vi "Main.vi"() -> ()   [LabVIEW 2020]
panel:
  out "Postać kanoniczna":string
  out "Max":dbl
  out "Min":dbl
  in  "Rząd pochodnej":i32=1 min=1 max=100
  out "string":string
  out "q":dbl
  out "p":dbl
  in  "start":dbl
  in  "end":dbl
  out "x3":string
  out "x2":string
  out "x1":string
  in  "równanie":bool
  in  "pochodna":bool
  in  "Liczby zespolone":bool
  out "Wykres":cluster{"Xaxis":dbl[], "f'(x)":dbl[]}[](graph)
  in  "x":dbl
  in  "f(x)":bool
  out "Wartość f(x)":dbl
  in  "stop":bool
  in  "d":dbl
  in  "c":dbl
  in  "b":dbl
  in  "a":dbl
  # "Podaj współczynniki:"
  # "Postać wzoru do podania: \n\nax^3 + bx^2 +cx +d =0"
  # "Zakres:"
  # "Współrzędne wierzchołka"
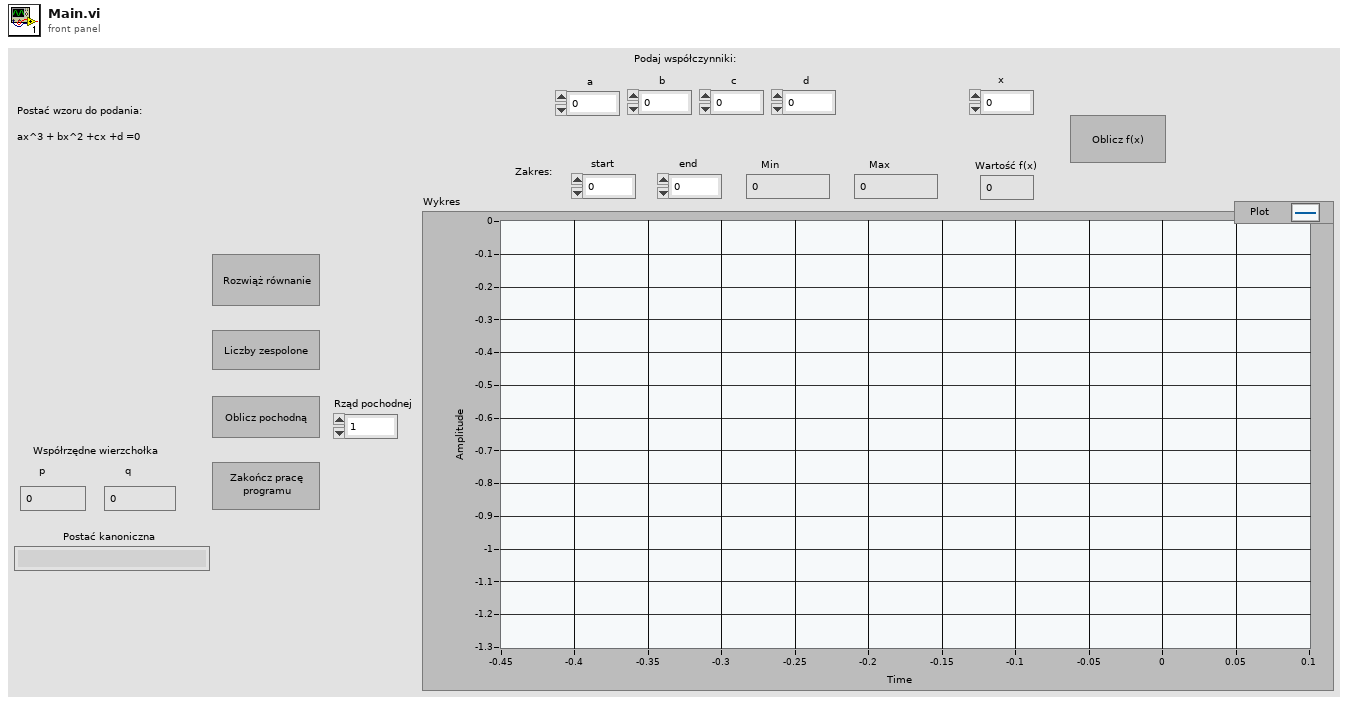
[diagram p1: front panel]
types:
  T1 = cluster{"współczynniki":cluster{"a":dbl, "b":dbl, "c":dbl, "d":dbl}, "x":dbl, "dFx":dbl[], "x2":cdb, "x3":cdb, "wsp. dFx":dbl[], "zespolone?":bool, "p":dbl, "q":dbl, "x[]":dbl[], "zakres":cluster{"od":dbl, "do":dbl}, "x1":cdb, "f(x)":dbl[], "stopień":enum16{"2", "3"}, "delta":i16, "Postać kanoniczna":string}
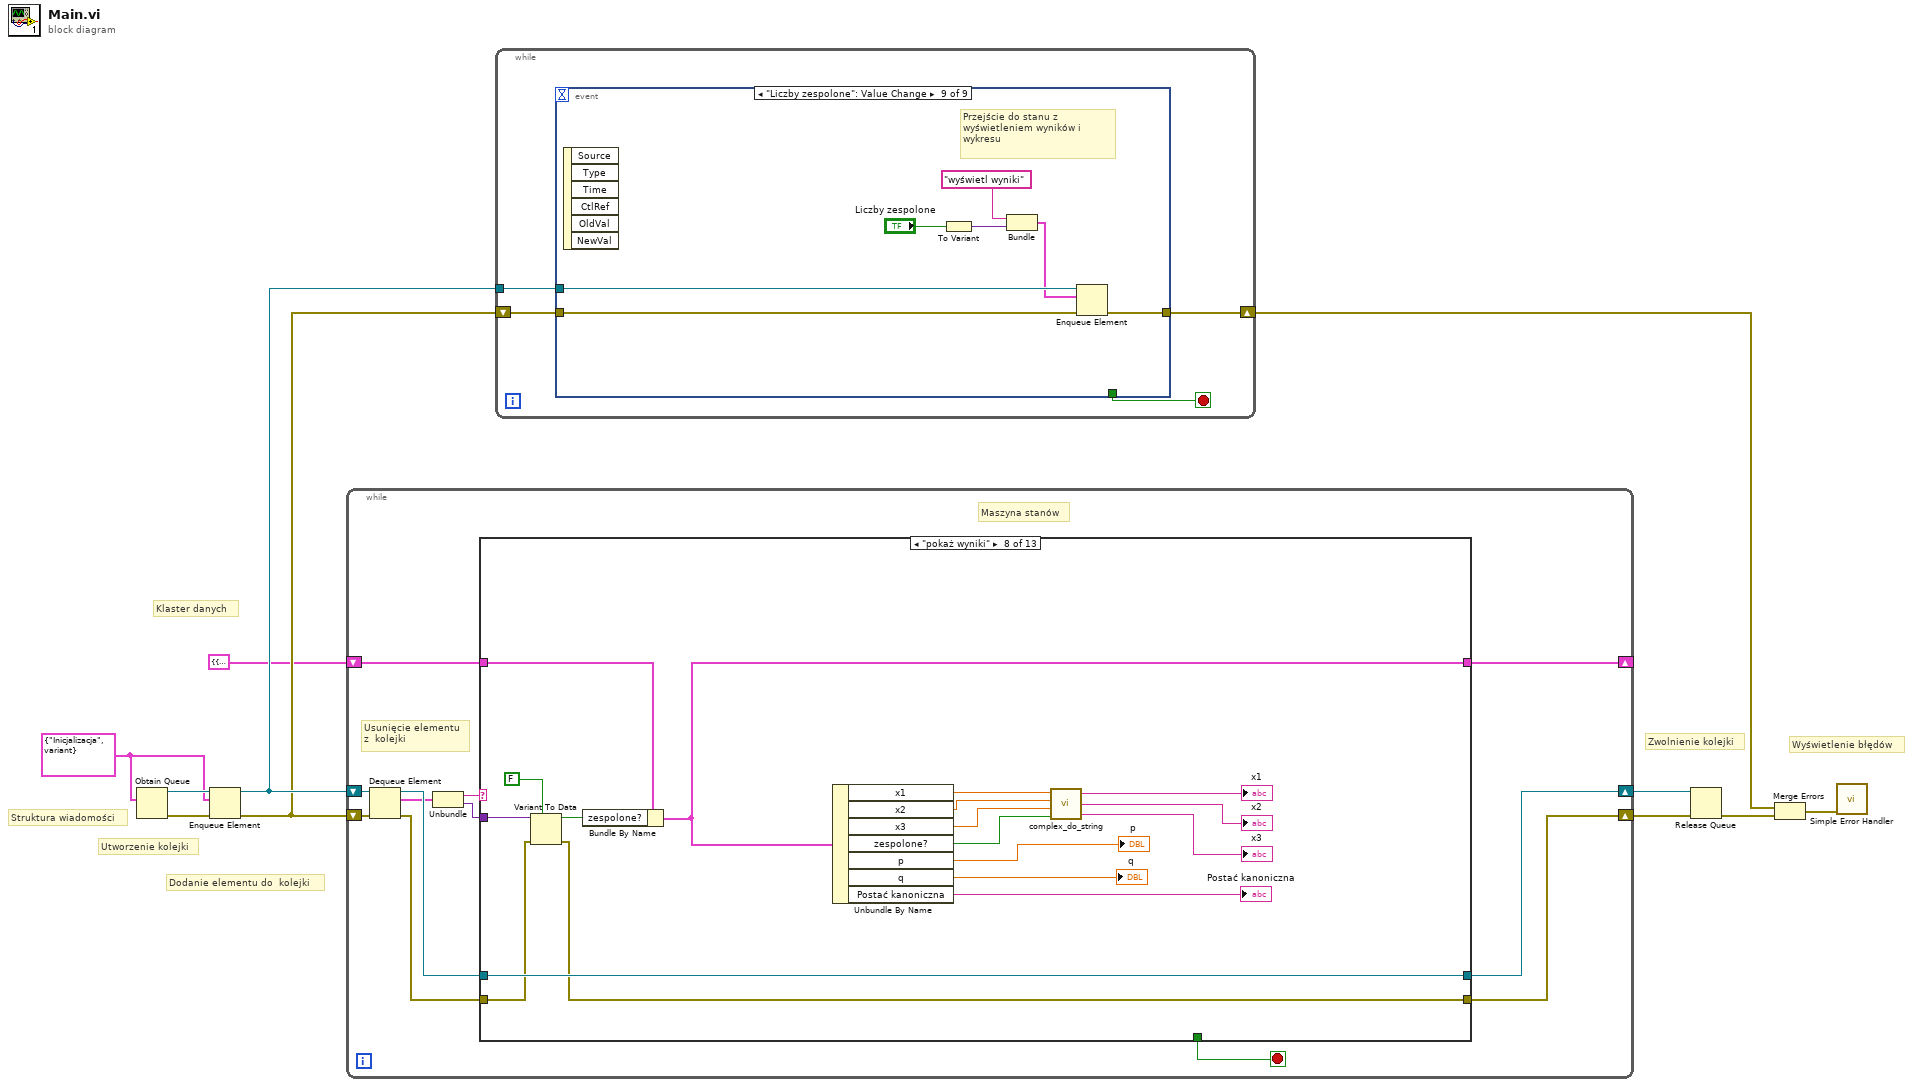
[diagram p0: block diagram]
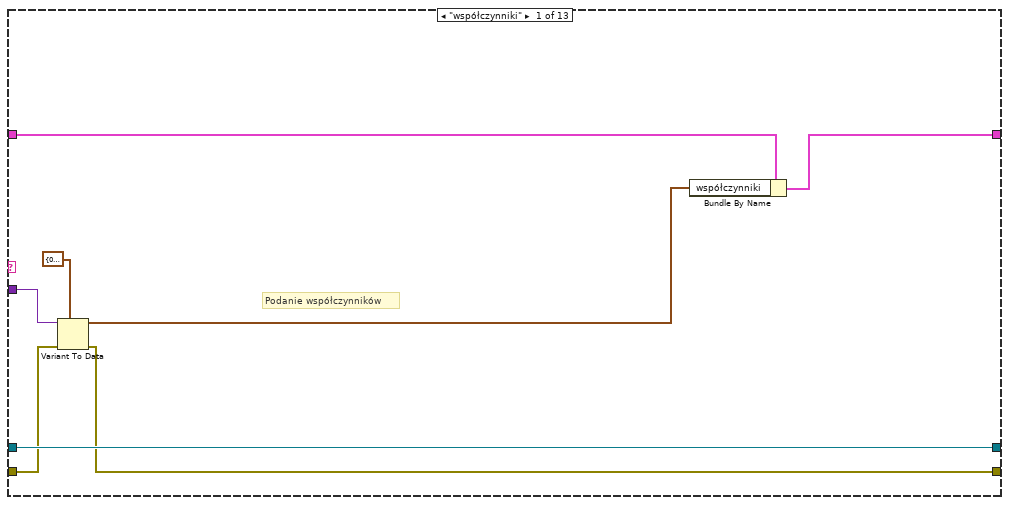
[diagram p2: hidden frame]
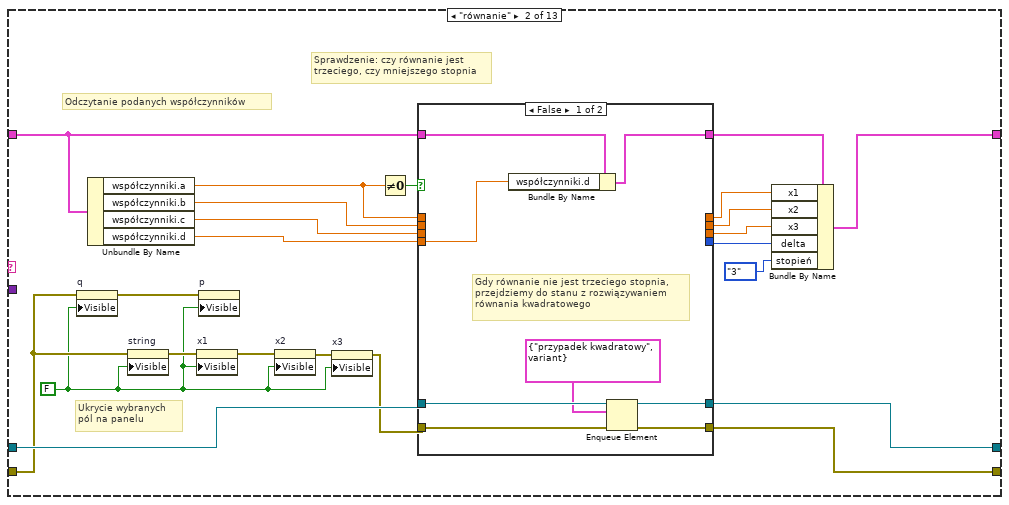
[diagram p3: hidden frame]
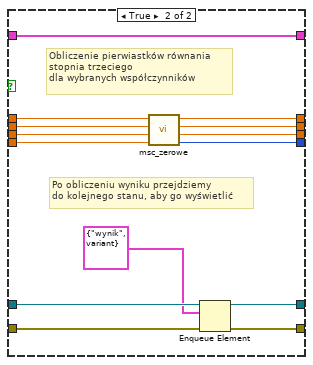
[diagram p4: hidden frame]
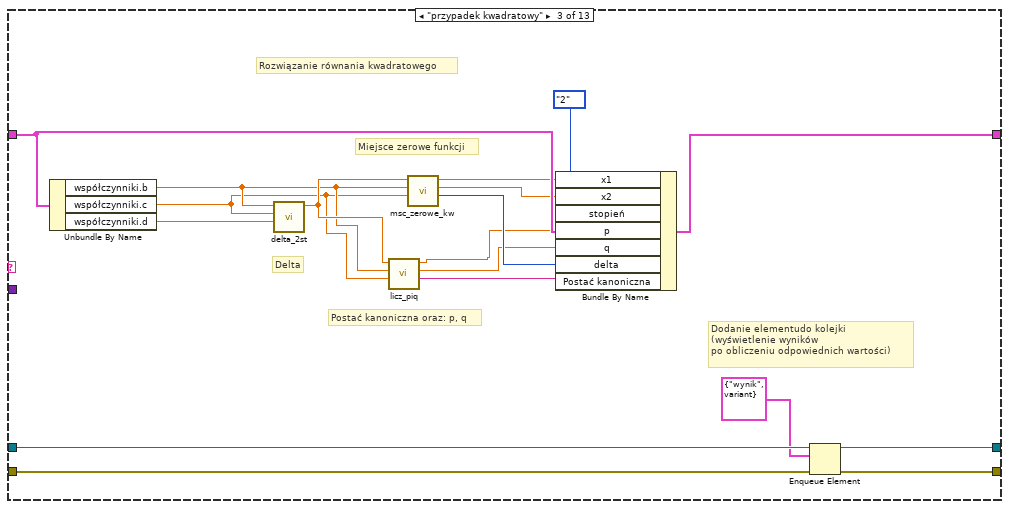
[diagram p5: hidden frame]
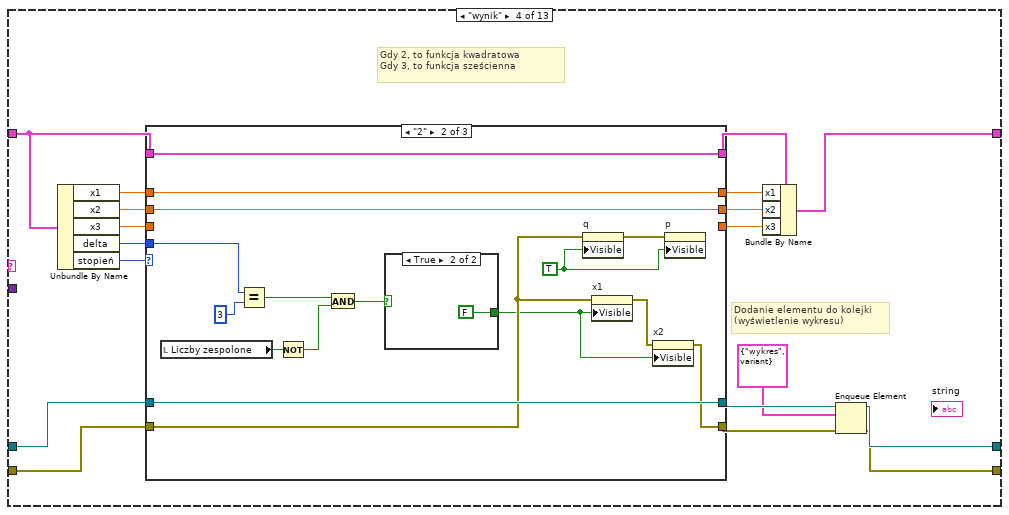
[diagram p6: hidden frame]
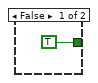
[diagram p8: hidden frame]
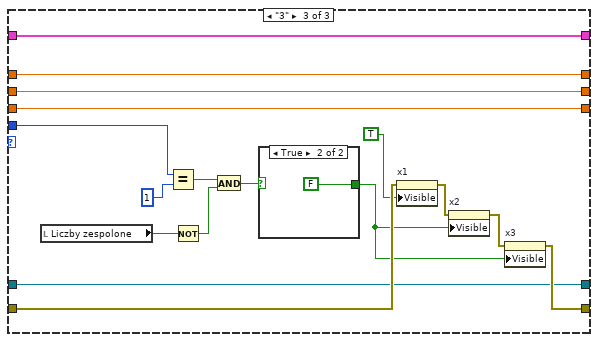
[diagram p9: hidden frame]
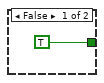
[diagram p10: hidden frame]
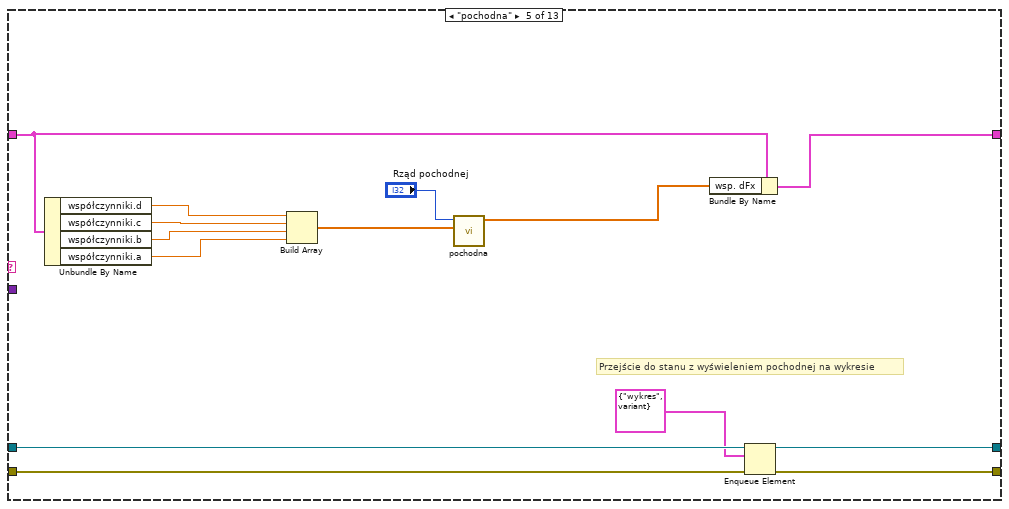
[diagram p11: hidden frame]
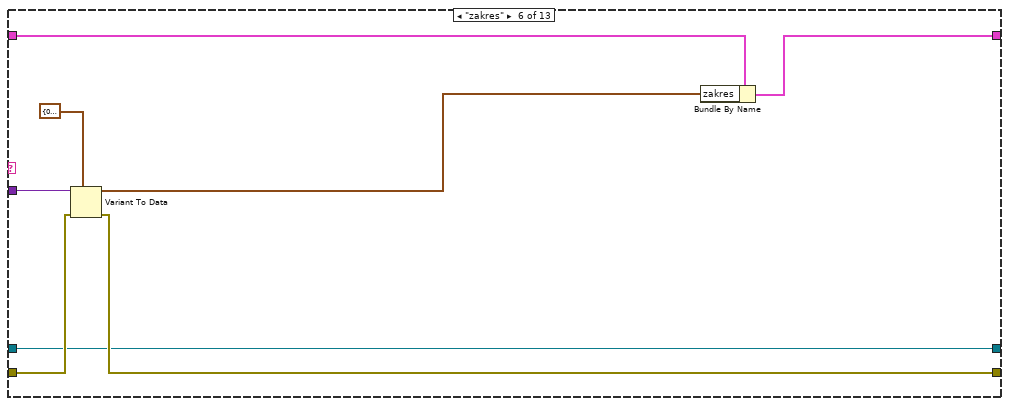
[diagram p12: hidden frame]
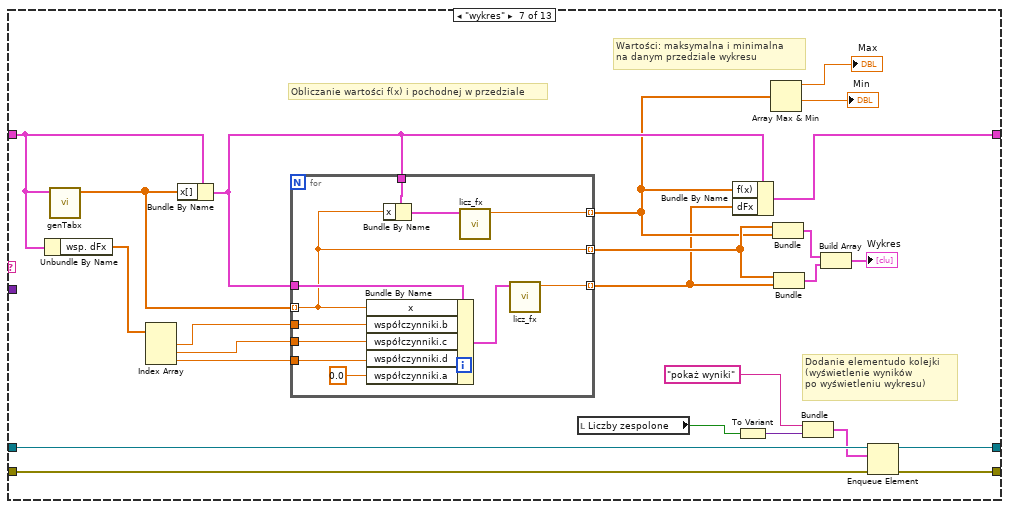
[diagram p13: hidden frame]
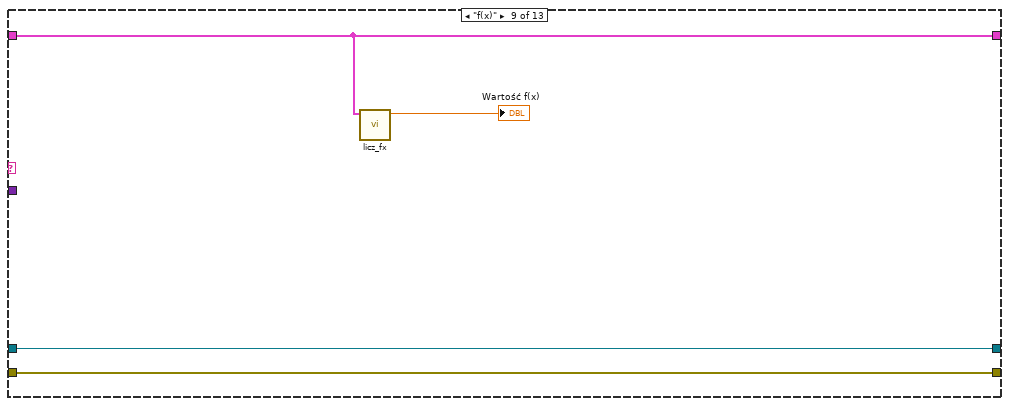
[diagram p14: hidden frame]
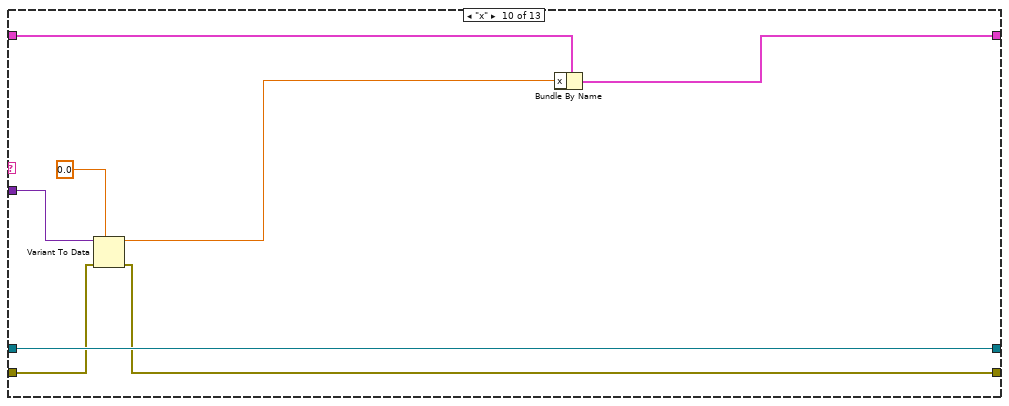
[diagram p15: hidden frame]
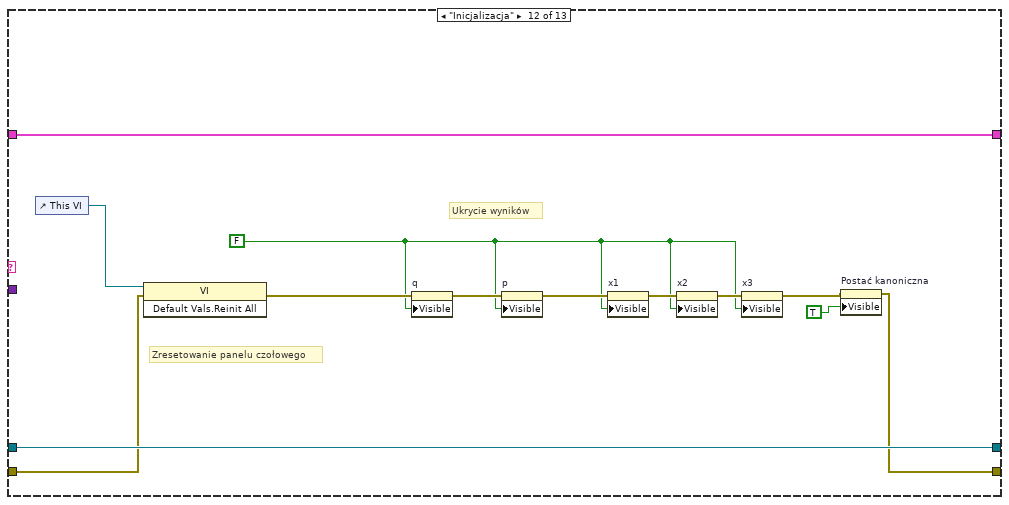
[diagram p17: hidden frame]
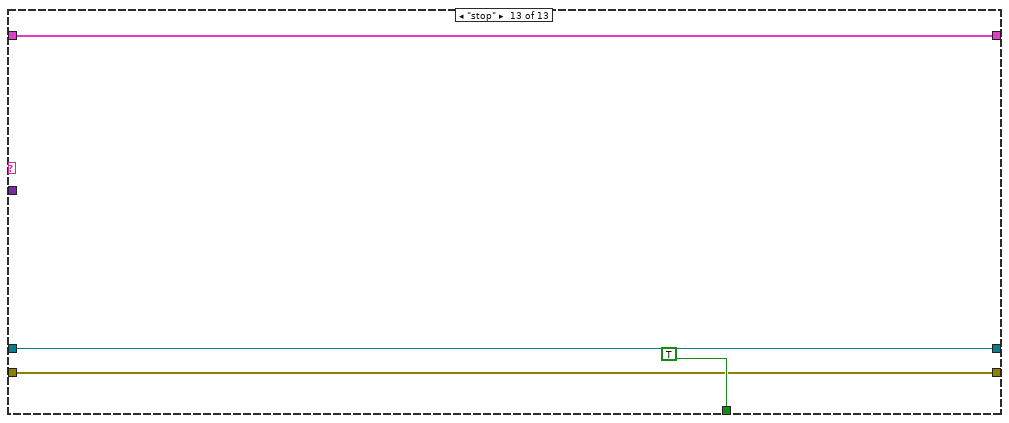
[diagram p18: hidden frame]
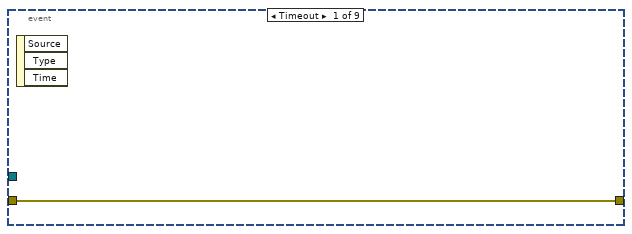
[diagram p19: hidden frame]
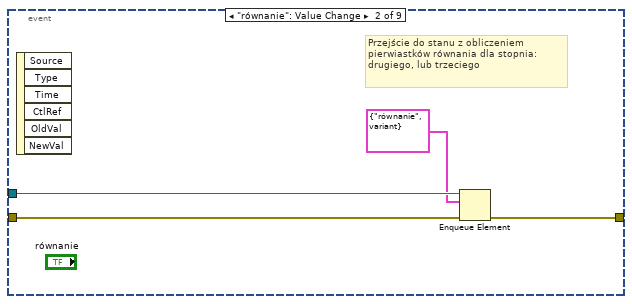
[diagram p20: hidden frame]
diagram:
  w9 = cluster{string, variant} {"Inicjalizacja", variant}
  # "Dodanie elementu do  kolejki"
  # "Struktura wiadomości"
  # "Wyświetlenie błędów"
  # "Zwolnienie kolejki"
  # "Klaster danych"
  # "Utworzenie kolejki"
  n1 = Obtain Queue(element data type=w9) -> (queue out=w11:refnum<queue>, error out=w10:errorcluster)  [unwired: 4 in, 1 out]
  n2 = Enqueue Element(queue=w11, element=w9, error in (no error)=w10) -> (queue out=w8:refnum<queue>, error out=w7:errorcluster)  [unwired: 1 in, 1 out]
  n3 = while {
    shift-right: [w12] -> _
    shift-left: T1 {"współczynniki"={"a"=0.0, "b"=0.0, "c"=0.0, "d"=0.0}, "x"=0.0, "dFx"=[], "x2"=0.0+0.0i, "x3"=0.0+0.0i, "wsp. dFx"=[], "zespolone?"=FALSE, "p"=0.0, "q"=0.0, "x[]"=[], "zakres"={"od"=0.0, "do"=0.0}, "x1"=0.0+0.0i, "f(x)"=[], "stopień"=enum."2", "delta"=0, "Postać kanoniczna"=""} -> [w15]
    shift-right: [w14] -> w4
    shift-left: w8 -> [w23]
    shift-right: [w13] -> w5
    shift-left: w7 -> [w22]
    stop <- w16 stop-if-true
    # "Usunięcie elementu\nz  kolejki"
    # "Maszyna stanów"
    n4 = Dequeue Element(queue=w23, error in (no error)=w22) -> (queue out=w21:refnum<queue>, element=w19:cluster{string, variant}, error out=w20:errorcluster)  [unwired: 1 in, 1 out]
    n5 = Unbundle(w19) -> (w18:string, w17:variant)
    n6 = case shown="\"pokaż wyniki\"" w18 {
      tunnel: w21 -> [w31 w49 w92 w111 w156 w167 w188 w223 w231 w239 w242 w255 w257]
      tunnel: w20 -> [w24 w35 w94 w112 w154 w173 w189 w219 w230 w235 w241 w252 w256]
      tunnel: w17 -> [w30 _ _ _ _ w174 _ w221 _ w238 _ _ _]
      tunnel: [_ _ _ _ _ _ _ _ _ _ _ _ TRUE] -> w16
      tunnel: w15 -> [w27 w48 w88 w103 w163 w170 w185 w222 w228 w234 w240 w254 w258]
      tunnel: [w28 w42 w89 w105 w165 w169 w198 w216 w228 w233 w240 w254 w258] -> w12
      tunnel: [w31 w34 w90 w109 w157 w167 w191 w223 w231 w239 w242 w255 w257] -> w14
      tunnel: [w25 w33 w91 w108 w155 w172 w190 w220 w230 w236 w241 w244 w256] -> w13
      frame "współczynniki" {
        # "Podanie współczynników"
        n7 = Variant To Data(error in=w24, type=cluster{"a":dbl, "b":dbl, "c":dbl, "d":dbl} {"a"=0.0, "b"=0.0, "c"=0.0, "d"=0.0} ("output cluster"), Variant=w30) -> (data=w26:cluster{"a":dbl, "b":dbl, "c":dbl, "d":dbl}, error out=w25:errorcluster)
        n8 = Bundle By Name(cluster=w27, "współczynniki"=w26) -> (w28:T1)
      }
      frame "równanie" {
        w32 = FALSE ("Visible")
        # "Ukrycie wybranych \npól na panelu"
        # "Sprawdzenie: czy równanie jest \ntrzeciego, czy mniejszego stopnia"
        # "Odczytanie podanych współczynników"
        n9 = property on="q" class="DigNum (strict)"(error in=w35, "Visible"=w32) -> (error out=w36:errorcluster)  [unwired: 1 in, 1 out]
        n10 = Unbundle By Name(w48) -> ("współczynniki.a"=w50:dbl, "współczynniki.b"=w53:dbl, "współczynniki.c"=w52:dbl, "współczynniki.d"=w54:dbl)
        n11 = property on="string" class="Str"(error in=w35, "Visible"=w32) -> (error out=w47:errorcluster)  [unwired: 1 in, 1 out]
        n12 = property on="x1" class="Str"(error in=w47, "Visible"=w32) -> (error out=w46:errorcluster)  [unwired: 1 in, 1 out]
        n13 = property on="p" class="DigNum (strict)"(error in=w36, "Visible"=w32) -> ()  [unwired: 1 in, 2 out]
        n14 = property on="x2" class="Str"(error in=w46, "Visible"=w32) -> (error out=w45:errorcluster)  [unwired: 1 in, 1 out]
        n15 = property on="x3" class="Str"(error in=w45, "Visible"=w32) -> (error out=w44:errorcluster)  [unwired: 1 in, 1 out]
        n16 = Not Equal To 0?(x=w50) -> (x != 0?=w51:bool)
        n17 = case shown="False" w51 {
          tunnel: w50 -> [_ w76]
          tunnel: w53 -> [_ w75]
          tunnel: w52 -> [_ w74]
          tunnel: w54 -> [w55 w73]
          tunnel: w49 -> [w62 w68]
          tunnel: [w61 w65] -> w34
          tunnel: [w60 w64] -> w33
          tunnel: w44 -> [w59 w66]
          tunnel: w48 -> [w57 w63]
          tunnel: [w56 w63] -> w43
          tunnel: [_ w72] -> w41
          tunnel: [_ w71] -> w40
          tunnel: [_ w70] -> w39
          tunnel: [_ w69] -> w37
          frame False {
            # "Gdy równanie nie jest trzeciego stopnia,\nprzejdziemy do stanu z rozwiązywaniem \nrównania kwadratowego"
            n18 = Bundle By Name(cluster=w57, "współczynniki.d"=w55) -> (w56:T1)
            n19 = Enqueue Element(queue=w62, element=cluster{string, variant} {"przypadek kwadratowy", variant}, error in (no error)=w59) -> (queue out=w61:refnum<queue>, error out=w60:errorcluster)  [unwired: 1 in, 1 out]
          }
          frame True {
            # "Obliczenie pierwiastków równania \nstopnia trzeciego \ndla wybranych współczynników"
            # "Po obliczeniu wyniku przejdziemy\ndo kolejnego stanu, aby go wyświetlić"
            n20 = call "msc_zerowe.vi"("d"=w73, "c"=w74, "b"=w75, "a"=w76) -> ("Ilość pierwiastków rzeczywistych"=w69:i16, "x3"=w70:cdb, "x2"=w71:cdb, "x1"=w72:cdb)  [unwired: 4 in]
            n21 = Enqueue Element(queue=w68, element=cluster{string, variant} {"wynik", variant}, error in (no error)=w66) -> (queue out=w65:refnum<queue>, error out=w64:errorcluster)  [unwired: 1 in, 1 out]
          }
        }
        n22 = Bundle By Name(cluster=w43, "x1"=w41, "x2"=w40, "x3"=w39, "delta"=w37, "stopień"=enum16{"2", "3"}."3") -> (w42:T1)
      }
      frame "przypadek kwadratowy" {
        # "Dodanie elementudo kolejki \n(wyświetlenie wyników \npo obliczeniu odpowiednich wartości)"
        # "Delta"
        # "Miejsce zerowe funkcji"
        # "Postać kanoniczna oraz: p, q"
        # "Rozwiązanie równania kwadratowego"
        n23 = Unbundle By Name(w88) -> ("współczynniki.b"=w81:dbl, "współczynniki.c"=w80:dbl, "współczynniki.d"=w93:dbl)
        n24 = call "delta_2st.vi"("c"=w93, "b"=w80, "a"=w81) -> ("Delta drugiego stopnia"=w82:dbl)  [unwired: 8 in]
        n25 = call "licz_piq.vi"("b"=w80, "a"=w81, "delta"=w82) -> ("Postać kanoniczna"=w77:string, "q"=w78:dbl, "p"=w79:dbl)  [unwired: 5 in]
        n26 = call "msc_zerowe_kw.vi"("b"=w80, "a"=w81, "delta"=w82) -> ("selector"=w83:i16, "x2"=w86:cdb, "x1"=w87:cdb)  [unwired: 6 in]
        n27 = Bundle By Name(cluster=w88, "x1"=w87, "x2"=w86, "stopień"=enum16{"2", "3"}."2", "p"=w79, "q"=w78, "delta"=w83, "Postać kanoniczna"=w77) -> (w89:T1)
        n28 = Enqueue Element(queue=w92, element=cluster{string, variant} {"wynik", variant}, error in (no error)=w94) -> (queue out=w90:refnum<queue>, error out=w91:errorcluster)  [unwired: 1 in, 1 out]
      }
      frame "wynik" {
        # "Dodanie elementu do kolejki \n(wyświetlenie wykresu)"
        # "Gdy 2, to funkcja kwadratowa\nGdy 3, to funkcja sześcienna"
        n29 = Unbundle By Name(w103) -> ("x1"=w102:cdb, "x2"=w101:cdb, "x3"=w97:cdb, "delta"=w95:i16, "stopień"=w96:enum16{"2", "3"})
        n30 = case shown="\"2\"" w96 {
          tunnel: [w115 w126 w140] -> w104
          tunnel: w103 -> [w115 w126 w140]
          tunnel: [w114 w131 w141] -> w107
          tunnel: w111 -> [w114 w131 w141]
          tunnel: w112 -> [w113 w118 w142]
          tunnel: [w113 w123 w145] -> w110
          tunnel: [_ w122 w137] -> w100
          tunnel: [_ w121 w136] -> w99
          tunnel: [_ _ w135] -> w98
          tunnel: w102 -> [_ w122 w137]
          tunnel: w101 -> [_ w121 w136]
          tunnel: w97 -> [_ _ w135]
          tunnel: w95 -> [_ w120 w134]
          frame Default {
          }
          frame "2" {
            w116 = TRUE ("Visible")
            n31 = local read "Liczby zespolone"() -> (w130:bool)
            n32 = Equal?(x=w120, y=i16 3) -> (x = y?=w129:bool)
            n33 = Not(x=w130) -> (.not. x?=w125:bool)
            n34 = And(x=w129, y=w125) -> (x .and. y?=w127:bool)
            n35 = case shown="True" w127 {
              tunnel: [TRUE ("Visible") FALSE ("Visible")] -> w117
              frame False {
              }
              frame True {
              }
            }
            n36 = property on="q" class="DigNum (strict)"(error in=w118, "Visible"=w116) -> (error out=w119:errorcluster)  [unwired: 1 in, 1 out]
            n37 = property on="x1" class="Str"(error in=w118, "Visible"=w117) -> (error out=w124:errorcluster)  [unwired: 1 in, 1 out]
            n38 = property on="x2" class="Str"(error in=w124, "Visible"=w117) -> (error out=w123:errorcluster)  [unwired: 1 in, 1 out]
            n39 = property on="p" class="DigNum (strict)"(error in=w119, "Visible"=w116) -> ()  [unwired: 1 in, 2 out]
          }
          frame "3" {
            n40 = local read "Liczby zespolone"() -> (w148:bool)
            n41 = Equal?(x=w134, y=i16 1) -> (x = y?=w150:bool)
            n42 = Not(x=w148) -> (.not. x?=w147:bool)
            n43 = And(x=w150, y=w147) -> (x .and. y?=w149:bool)
            n44 = case shown="True" w149 {
              tunnel: [TRUE ("Visible") FALSE ("Visible")] -> w139
              frame False {
              }
              frame True {
              }
            }
            n45 = property on="x1" class="Str"(error in=w142, "Visible"=TRUE) -> (error out=w143:errorcluster)  [unwired: 1 in, 1 out]
            n46 = property on="x2" class="Str"(error in=w143, "Visible"=w139) -> (error out=w144:errorcluster)  [unwired: 1 in, 1 out]
            n47 = property on="x3" class="Str"(error in=w144, "Visible"=w139) -> (error out=w145:errorcluster)  [unwired: 1 in, 1 out]
          }
        }
        n48 = Bundle By Name(cluster=w104, "x1"=w100, "x2"=w99, "x3"=w98) -> (w105:T1)
        n49 = Enqueue Element(queue=w107, element=cluster{string, variant} {"wykres", variant}, error in (no error)=w110) -> (queue out=w109:refnum<queue>, error out=w108:errorcluster)  [unwired: 1 in, 1 out]
      }
      frame "pochodna" {
        # "Przejście do stanu z wyświeleniem pochodnej na wykresie"
        n50 = Unbundle By Name(w163) -> ("współczynniki.d"=w162:dbl, "współczynniki.c"=w161:dbl, "współczynniki.b"=w160:dbl, "współczynniki.a"=w159:dbl)
        n51 = Build Array(w162, w161, w160, w159) -> (w158:dbl[])
        n52 = call "pochodna.vi"("współczynniki"=w158, "rząd"="Rząd pochodnej") -> ("pochodna"=w164:dbl[])  [unwired: 9 in]
        n53 = Bundle By Name(cluster=w163, "wsp. dFx"=w164) -> (w165:T1)
        n54 = Enqueue Element(queue=w156, element=cluster{string, variant} {"wykres", variant}, error in (no error)=w154) -> (queue out=w157:refnum<queue>, error out=w155:errorcluster)  [unwired: 1 in, 1 out]
      }
      frame "zakres" {
        n55 = Variant To Data(error in=w173, type=cluster{"od":dbl, "do":dbl} {"od"=0.0, "do"=0.0} ("output cluster"), Variant=w174) -> (data=w168:cluster{"od":dbl, "do":dbl}, error out=w172:errorcluster)
        n56 = Bundle By Name(cluster=w170, "zakres"=w168) -> (w169:T1)
      }
      frame "wykres" {
        # "Wartości: maksymalna i minimalna \nna danym przedziale wykresu"
        # "Dodanie elementudo kolejki \n(wyświetlenie wyników \npo wyświetleniu wykresu)"
        # "Obliczanie wartości f(x) i pochodnej w przedziale"
        n57 = Unbundle By Name(w185) -> ("wsp. dFx"=w195:dbl[])
        n58 = call "genTabx.vi"("Cluster"=w185) -> ("Ramp Pattern"=w186:dbl[])  [unwired: 10 in]
        n59 = Index Array(array=w195) -> (element #1=w194:dbl, element #2=w193:dbl, element #3=w192:dbl)  [unwired: 3 in]
        n60 = Bundle By Name(cluster=w185, "x[]"=w186) -> (w187:T1)
        n61 = for {
          tunnel: w187 -> [w209]
          tunnel: w186 -> [w199] mode=indexing
          tunnel: [w208] -> w180 mode=indexing
          tunnel: w194 -> [w207]
          tunnel: w193 -> [w206]
          tunnel: w192 -> [w205]
          tunnel: w187 -> [w201]
          tunnel: [w200] -> w181 mode=indexing
          tunnel: [w199] -> w182 mode=indexing
          n62 = Bundle By Name(cluster=w209, "x"=w199, "współczynniki.b"=w207, "współczynniki.c"=w206, "współczynniki.d"=w205, "współczynniki.a"=0.0 ("Coefficients.a")) -> (w203:T1)
          n63 = Bundle By Name(cluster=w201, "x"=w199) -> (w202:T1)
          n64 = call "licz_fx.vi"("Cluster"=w202) -> ("f(x)"=w200:dbl)  [unwired: 10 in]
          n65 = call "licz_fx.vi"("Cluster"=w203) -> ("f(x)"=w208:dbl)  [unwired: 10 in]
        }
        n66 = local read "Liczby zespolone"() -> (w176:bool)
        n67 = Bundle By Name(cluster=w187, "f(x)"=w181, "dFx"=w180) -> (w198:T1)
        n68 = To Variant(anything=w176) -> (Variant=w175:variant)
        n69 = Array Max & Min(array=w181) -> (max value=→"Max":dbl, min value=→"Min":dbl)  [unwired: 2 out]
        n70 = Bundle(w182, w181) -> (w183:cluster{dbl[], dbl[]})  [unwired: 1 in]
        n71 = Bundle(w182, w180) -> (w184:cluster{dbl[], dbl[]})  [unwired: 1 in]
        n72 = Bundle("pokaż wyniki", "Variant"=w175) -> (w178:cluster{string, "Variant":variant})  [unwired: 1 in]
        n73 = Build Array(w183, w184) -> (→"Wykres":cluster{dbl[], dbl[]}[])
        n74 = Enqueue Element(queue=w188, element=w178, error in (no error)=w189) -> (queue out=w191:refnum<queue>, error out=w190:errorcluster)  [unwired: 1 in, 1 out]
      }
      frame "pokaż wyniki" {
        n75 = Variant To Data(error in=w219, type=FALSE, Variant=w221) -> (data=w217:bool, error out=w220:errorcluster)
        n76 = Bundle By Name(cluster=w222, "zespolone?"=w217) -> (w216:T1)
        n77 = Unbundle By Name(w216) -> ("x1"=w227:cdb, "x2"=w226:cdb, "x3"=w225:cdb, "zespolone?"=w224:bool, "p"=→"p":dbl, "q"=→"q":dbl, "Postać kanoniczna"=→"Postać kanoniczna":string)
        n78 = call "complex_do_string.vi"("Czy zespolone"=w224, "x3"=w225, "x2"=w226, "x1"=w227) -> ("x3"=→"x3":string, "x2"=→"x2":string, "x1"=→"x1":string)
      }
      frame "f(x)" {
        n79 = call "licz_fx.vi"("Cluster"=w228) -> ("f(x)"=→"Wartość f(x)":dbl)  [unwired: 10 in]
      }
      frame "x" {
        n80 = Variant To Data(error in=w235, type=0.0 ("Watrość x ="), Variant=w238) -> (data=w232:dbl, error out=w236:errorcluster)
        n81 = Bundle By Name(cluster=w234, "x"=w232) -> (w233:T1)
      }
      frame Default {
      }
      frame "Inicjalizacja" {
        w245 = FALSE ("Visible")
        # "Ukrycie wyników"
        # "Zresetowanie panelu czołowego"
        n82 = control-ref of="This VI"() -> (w253:refnum<vi>)
        n83 = invoke class="VI" method="Default Vals.Reinit All"(reference=w253, error in=w252) -> (error out=w248:errorcluster)  [unwired: 1 in, 2 out]
        n84 = property on="q" class="DigNum (strict)"(error in=w248, "Visible"=w245) -> (error out=w249:errorcluster)  [unwired: 1 in, 1 out]
        n85 = property on="p" class="DigNum (strict)"(error in=w249, "Visible"=w245) -> (error out=w247:errorcluster)  [unwired: 1 in, 1 out]
        n86 = property on="x1" class="Str"(error in=w247, "Visible"=w245) -> (error out=w251:errorcluster)  [unwired: 1 in, 1 out]
        n87 = property on="x2" class="Str"(error in=w251, "Visible"=w245) -> (error out=w250:errorcluster)  [unwired: 1 in, 1 out]
        n88 = property on="x3" class="Str"(error in=w250, "Visible"=w245) -> (error out=w246:errorcluster)  [unwired: 1 in, 1 out]
        n89 = property on="Postać kanoniczna" class="Str"(error in=w246, "Visible"=TRUE) -> (error out=w244:errorcluster)  [unwired: 1 in, 1 out]
      }
      frame "stop" {
      }
    }
  }
  n90 = while {
    tunnel: w8 -> [w260]
    shift-right: [w262] -> w2
    shift-left: w7 -> [w261]
    stop <- w263 stop-if-true
    n91 = event shown="[8] \"Liczby zespolone\": Value Change" {
      selector: _ -> [_ _ _ _ _ _ _ _ _]
      dyn-events: _ -> [_ _ _ _ _ _ _ _ _]
      timeout: _ -> [_ _ _ _ _ _ _ _ _]
      tunnel: [_ _ _ _ _ _ TRUE _ _] -> w263
      tunnel: [w264 w267 w277 w281 w287 w294 w300 w308 w314] -> w262
      tunnel: w261 -> [w264 w268 w275 w280 w288 w296 w299 w306 w315]
      tunnel: w260 -> [_ w266 w276 w279 w286 w295 w298 w307 w313]
      event Timeout {
        n92 = event-data() -> ()  [unwired: 1 in, 3 out]
      }
      event "równanie": Value Change {
        # "Przejście do stanu z obliczeniem pierwiastków równania dla stopnia: drugiego, lub trzeciego"
        n93 = event-data() -> ()  [unwired: 1 in, 6 out]
        n94 = Enqueue Element(queue=w266, element=cluster{string, variant} {"równanie", variant}, error in (no error)=w268) -> (error out=w267:errorcluster)  [unwired: 1 in, 2 out]
      }
      event "start", "end": Value Change {
        # "Odczytanie zakresu wartości: x dla wykresu funkcji"
        n95 = event-data() -> ()  [unwired: 1 in, 6 out]
        n96 = Bundle("start"="start", "end"="end") -> (w271:cluster{"start":dbl, "end":dbl})  [unwired: 1 in]
        n97 = To Variant(anything=w271) -> (Variant=w272:variant)
        n98 = Bundle("zakres", "Variant"=w272) -> (w274:cluster{string, "Variant":variant})  [unwired: 1 in]
        n99 = Enqueue Element(queue=w276, element=w274, error in (no error)=w275) -> (error out=w277:errorcluster)  [unwired: 1 in, 2 out]
      }
      event "pochodna": Value Change {
        n100 = event-data() -> ()  [unwired: 1 in, 6 out]
        n101 = Enqueue Element(queue=w279, element=cluster{string, variant} {"pochodna", variant}, error in (no error)=w280) -> (error out=w281:errorcluster)  [unwired: 1 in, 2 out]
      }
      event "a", "b", "c", "d": Value Change {
        # "Przejście do stanu z podaniem\ni wczytaniem współczynników"
        n102 = event-data() -> ()  [unwired: 1 in, 6 out]
        n103 = Bundle("a"="a", "b"="b", "c"="c", "d"="d") -> (w283:cluster{"a":dbl, "b":dbl, "c":dbl, "d":dbl})  [unwired: 1 in]
        n104 = To Variant(anything=w283) -> (Variant=w282:variant)
        n105 = Bundle("współczynniki", "Variant"=w282) -> (w285:cluster{string, "Variant":variant})  [unwired: 1 in]
        n106 = Enqueue Element(queue=w286, element=w285, error in (no error)=w288) -> (error out=w287:errorcluster)  [unwired: 1 in, 2 out]
      }
      event "f(x)": Value Change {
        # "Przejście do stanu z \nobliczeniem wartości funkcji"
        n107 = event-data() -> ()  [unwired: 1 in, 6 out]
        n108 = Enqueue Element(queue=w295, element=cluster{string, variant} {"f(x)", variant}, error in (no error)=w296) -> (error out=w294:errorcluster)  [unwired: 1 in, 2 out]
      }
      event "stop": Value Change {
        # "Koniec pracy programu"
        n109 = event-data() -> ()  [unwired: 1 in, 6 out]
        n110 = Enqueue Element(queue=w298, element=cluster{string, variant} {"stop", variant}, error in (no error)=w299) -> (error out=w300:errorcluster)  [unwired: 1 in, 2 out]
      }
      event "x": Value Change {
        # "Przejście do stanu z \npodaniem wartości: x"
        n111 = event-data() -> ()  [unwired: 1 in, 6 out]
        n112 = To Variant(anything="x") -> (Variant=w302:variant)
        n113 = Bundle("x", "Variant"=w302) -> (w305:cluster{string, "Variant":variant})  [unwired: 1 in]
        n114 = Enqueue Element(queue=w307, element=w305, error in (no error)=w306) -> (error out=w308:errorcluster)  [unwired: 1 in, 2 out]
      }
      event "Liczby zespolone": Value Change {
        # "Przejście do stanu z \nwyświetleniem wyników i wykresu"
        n115 = event-data() -> ()  [unwired: 1 in, 6 out]
        n116 = To Variant(anything="Liczby zespolone") -> (Variant=w309:variant)
        n117 = Bundle("wyświetl wyniki", "Variant"=w309) -> (w311:cluster{string, "Variant":variant})  [unwired: 1 in]
        n118 = Enqueue Element(queue=w313, element=w311, error in (no error)=w315) -> (error out=w314:errorcluster)  [unwired: 1 in, 2 out]
      }
    }
  }
  n119 = Release Queue(queue=w4, error in (no error)=w5) -> (error out=w3:errorcluster)  [unwired: 1 in, 2 out]
  n120 = Merge Errors(w2, w3) -> (w1:errorcluster)
  n121 = call <vilib>:"Simple Error Handler.vi"("error in (no error)"=w1) -> ()  [unwired: 4 in, 5 out]
